vi "Excel - Convert Column to Index (James).vi"(11 "Column Name in":string) -> (3 "Column Index out":i32)   [LabVIEW 2014]
doc: "Converts column name from excel's format to an index.\n\nEx: \"A\" -> 0\n \"AA\" -> 26\n \"AB\" -> 27"
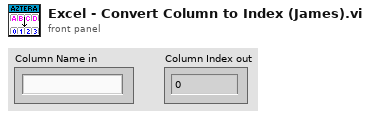
[diagram p1: front panel]
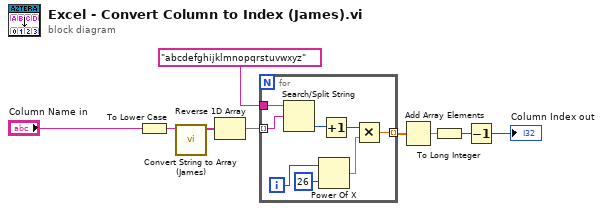
[diagram p0: block diagram]
diagram:
  n1 = To Lower Case(string="Column Name in") -> (all lower case string=w2:string)
  n2 = call "Convert String to Array (James).vi"("String in"=w2) -> ("Array out"=w1:string[])  [unwired: 9 in, 1 out]
  n3 = Reverse 1D Array(array=w1) -> (reversed array=w4:string[])
  n4 = for {
    tunnel: w4 -> [w16] mode=indexing
    tunnel: "abcdefghijklmnopqrstuvwxyz" ("String") -> [w17]
    tunnel: [w10] -> w6 mode=indexing
    i -> [w12]
    n5 = Search/Split String(string=w17, search string/char (-)=w16) -> (offset of match=w15:i32)  [unwired: 1 in, 2 out]
    n6 = Power Of X(1:26 ("x"), 2:w12) -> (0:w11:dbl)
    n7 = Increment(x=w15) -> (x+1=w14:i32)
    n8 = Multiply(x=w14, y=w11) -> (x*y=w10:dbl)
  }
  n9 = Add Array Elements(numeric array=w6) -> (sum=w7:dbl)
  n10 = To Long Integer(number=w7) -> (32bit integer=w8:i32)
  n11 = Decrement(x=w8) -> (x-1=→"Column Index out":i32)
